vi "NI6602.Read.vi"(0 "i ref in":refnum<vi>, 5 "error in (no error)":errorcluster) -> (14 "i ref out":refnum<vi>, 19 "error out":errorcluster)   [LabVIEW 2014, in "NI6602.lvlib"]
doc: "Reads out the counter and sets the Integral as well as the Rate Values.\n\nLicense Agreement for this software:\n\nCopyright (C)\nGesellschaft für Schwerionenforschung, GSI\nPlanckstr. 1\n64291 Darmstadt\nGermany\n\nContact: D.Beck@gsi.de \n\nThis program is free software; you can redistribute it and/or modify it under the terms of the \nGNU General Public License as published by the Free Software Foundation; either version 2 of \nthe license, or (at your option) any later version.\n\nThis program is distributed in the hope that it will be useful, but WITHOUT ANY WARRANTY; \nwithout even the implied warranty of MERCHANTABILITY or FITNESS FOR A PARTICULAR PURPOSE. See the GNU General License for more details (http://www.gnu.org).\n\nGesellschaft für Schwerionenforschung, GSI\nPlanckstr. 1, 64291 Darmstadt, Germany\nFor all questions and ideas contact: M.Richter@gsi.de, H.Brand@gsi.de or D.Beck@gsi.de.\nLast update: 16-JUN-2004"
uses:
  NI6602.lvlib
  CSlibraries-extern/DimLVEvent/LVDimInterface/LVDimInterface.lvlib
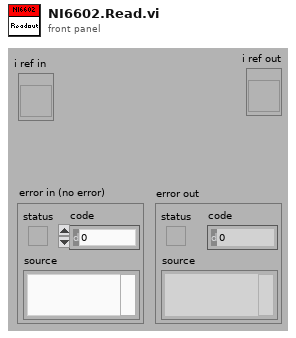
[diagram p1: front panel]
types:
  T1 = typedef "NI6602.lvlib/NI6602.i attribute.ctl" = cluster{"CounterDAQ Channels":cluster{"task":refnum<k21>, "Channel Name":string}[], "RateServiceIDs":i32[], "Running?":bool, "IntegralServiceIDs":i32[], "ThresholdID":i32, "Threshold":dbl, "IntegralValues":dbl[], "Stopped?":bool}
  T2 = cluster{"task":refnum<k21>, "Channel Name":string}[]
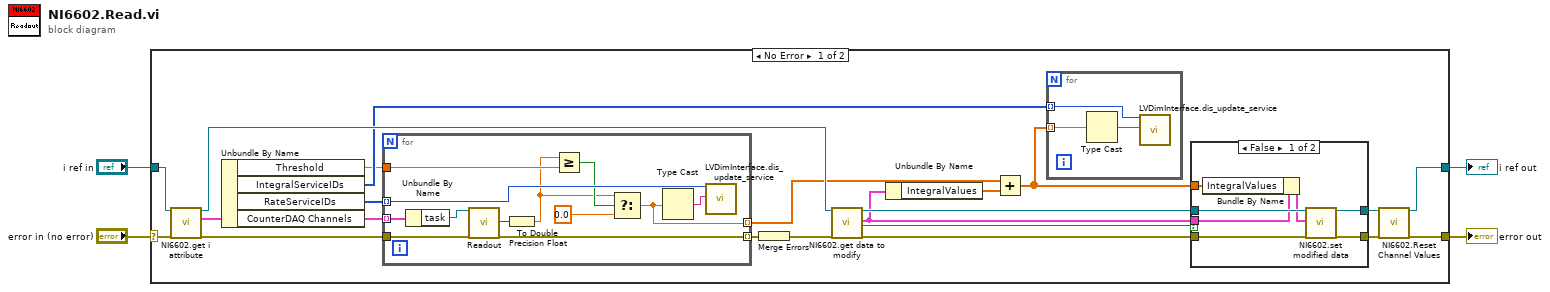
[diagram p0: block diagram]
diagram:
  n1 = case shown="No Error" "error in (no error)" {
    selector: "error in (no error)" -> [w25 w52]
    tunnel: [w19 w51] -> w4
    tunnel: [w18 w52] -> w3
    tunnel: "i ref in" -> [w23 w51]
    frame No Error {
      n2 = call "NI6602.get i attribute.vi"("i ref in"=w23, "error in (no error)"=w25) -> ("i ref out"=w14:refnum<vi>, "i attribute"=w22:T1, "error out"=w24:errorcluster)  [unwired: 15 in]
      n3 = Unbundle By Name(w22) -> ("Threshold"=w5:dbl, "IntegralServiceIDs"=w6:i32[], "RateServiceIDs"=w20:i32[], "CounterDAQ Channels"=w21:T2)
      n4 = for {
        tunnel: w24 -> [w50]
        tunnel: [w49] -> w26 mode=indexing
        tunnel: w21 -> [w48] mode=indexing
        tunnel: w20 -> [w46] mode=indexing
        tunnel: [w40] -> w8 mode=indexing
        tunnel: w5 -> [w43]
        n5 = Unbundle By Name(w48) -> ("task"=w47:refnum<k21>)
        n6 = call "Readout.vi"("task/channels in"=w47, "error in"=w50) -> ("data"=w44:u32, "error out"=w49:errorcluster)  [unwired: 15 in, 1 out]
        n7 = To Double Precision Float(number=w44) -> (double precision float=w41:dbl)
        n8 = Greater Or Equal?(x=w41, y=w43) -> (x >= y?=w42:bool)
        n9 = Select(t=w41, s=w42, f=0.0) -> (s? t:f=w40:dbl)
        n10 = Type Cast(x=w40) -> (*(type *) &x=w45:string)  [unwired: 1 in]
        n11 = call "LVDimInterface.dis_update_service.vi"("my_serviceID"=w46, "data"=w45) -> ()  [unwired: 15 in, 3 out]
      }
      n12 = Merge Errors(w26) -> (w17:errorcluster)
      n13 = call "NI6602.get data to modify.vi"("i ref in"=w14, "error in (no error)"=w17) -> ("i ref out"=w13:refnum<vi>, "i attribute"=w10:T1, "timed out"=w11:bool, "error out"=w16:errorcluster)  [unwired: 14 in]
      n14 = Unbundle By Name(w10) -> ("IntegralValues"=w9:dbl[])
      n15 = Add(x=w8, y=w9) -> (x+y=w7:dbl[])
      n16 = for {
        tunnel: w7 -> [w28] mode=indexing
        tunnel: w6 -> [w27] mode=indexing
        n17 = Type Cast(x=w28) -> (*(type *) &x=w29:string)  [unwired: 1 in]
        n18 = call "LVDimInterface.dis_update_service.vi"("my_serviceID"=w27, "data"=w29) -> ()  [unwired: 15 in, 3 out]
      }
      n19 = case shown="False" w11 {
        tunnel: w16 -> [w36 w37]
        tunnel: [w35 w37] -> w15
        tunnel: w13 -> [w34 w38]
        tunnel: [w33 w38] -> w12
        tunnel: w10 -> [w31 _]
        tunnel: w7 -> [w30 _]
        frame False {
          n20 = Bundle By Name(cluster=w31, "IntegralValues"=w30) -> (w32:T1)
          n21 = call "NI6602.set modified data.vi"("i ref in"=w34, "i attribute"=w32, "error in (no error)"=w36) -> ("i ref out"=w33:refnum<vi>, "error out"=w35:errorcluster)  [unwired: 15 in]
        }
        frame True {
        }
      }
      n22 = call "NI6602.Reset Channel Values.vi"("i ref in"=w12, "error in (no error)"=w15) -> ("i ref out"=w19:refnum<vi>, "error out"=w18:errorcluster)  [unwired: 16 in]
    }
    frame Error {
    }
  }
  "i ref out" <- w4
  "error out" <- w3
